vi "Acquire voltage waveform.vi"(5 "channel index":i8, 7 "Sample rate":dbl format="%.2f", 11 "data points to acquire":u32=1000 min=1) -> (6 "channel data array":sgl[](array[numeric]) format="%.5f", 8 "mean":dbl format="%.2f", 10 "cv":dbl format="%.2f", 14 "canceled":bool)   [LabVIEW 2015]
uses:
  DAQ configuration/Sensor buffer command.ctl
  <vilib>/Analysis/NI_AALBase.lvlib
panel:
  in  "Monitoring sample":bool
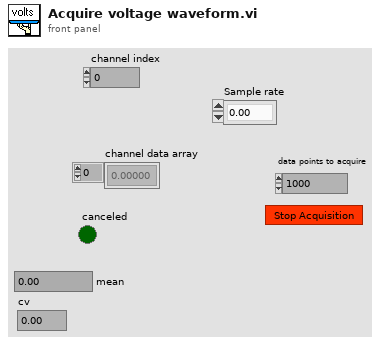
[diagram p1: front panel]
types:
  T1 = typedef "Sensor buffer command.ctl" = enum16{"read average", "read recent", "read all", "write", "set buffer size", "Read channel config", "Write channel config", "clear"}
  T2 = typedef "Sensor data.ctl" = cluster{" Sensor array":T3[], "Time":dbl}
  T3 = typedef "sensor cluster.ctl" = cluster{"voltage":sgl, "scaled":sgl, "units":string, "Out of Range":bool}
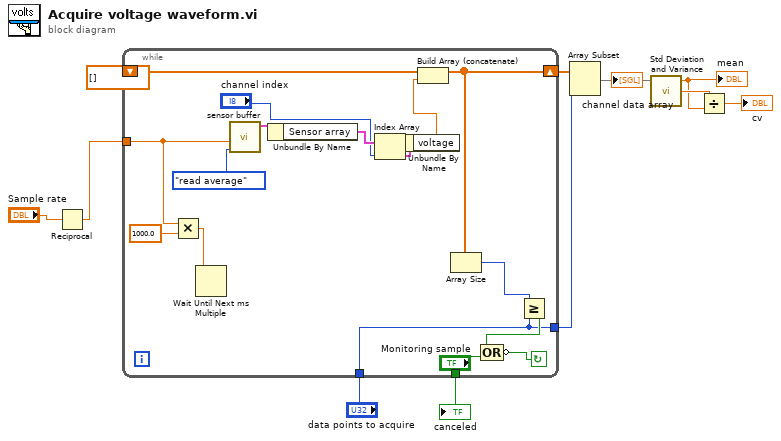
[diagram p0: block diagram]
diagram:
  n1 = Reciprocal(x="Sample rate") -> (1/x=w1:dbl)
  n2 = while {
    tunnel: "data points to acquire" -> [w21]
    tunnel: [w21] -> w4
    tunnel: ["Monitoring sample"] -> w8
    shift-left: sgl[] [] -> [w24]
    shift-right: [w22] -> w6
    tunnel: w1 -> [w14]
    stop <- w27 continue-if-true
    n3 = Multiply(x=w14, y=1000.0) -> (x*y=w12:dbl)
    n4 = Wait Until Next ms Multiple(millisecond multiple=w12) -> ()  [unwired: 1 out]
    n5 = call "sensor buffer.vi"("command"=Sensor_buffer_command."read average", "smooth interval (s)"=w14) -> ("Calibrated data"=w20:T2)  [unwired: 5 in, 4 out]
    n6 = Unbundle By Name(w20) -> ("Sensor array"=w19:T3[])
    n7 = Index Array(array=w19, index="channel index") -> (element=w17:T3)
    n8 = Unbundle By Name(w17) -> ("voltage"=w16:sgl)
    n9 = Build Array (concatenate)(w24, w16) -> (w22:sgl[])
    n10 = Array Size(array=w22) -> (size(s)=w23:i32)
    n11 = Greater Or Equal?(x=w23, y=w21) -> (x >= y?=w25:bool)
    n12 = Compound Arithmetic op=OR(w25, "Monitoring sample") -> (invert w27:bool)
  }
  "canceled" <- w8
  n13 = Array Subset(array=w6, length=w4) -> (w7:sgl[])  [unwired: 1 in]
  "channel data array" <- w7
  n14 = call <vilib>:"Std Deviation and Variance.vi"("X"=w7) -> ("mean"=w10:dbl, "standard deviation"=w11:dbl)  [unwired: 1 in, 1 out]
  "mean" <- w10
  n15 = Divide(x=w11, y=w10) -> (x/y=→"cv":dbl)
